vi "proc_checkErrors.vi"(1 "handle":i32) -> (0 "return value":i32)   [LabVIEW 2010]
uses:
  lib/MWT.dll
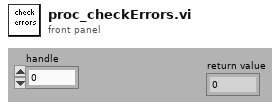
[diagram p1: front panel]
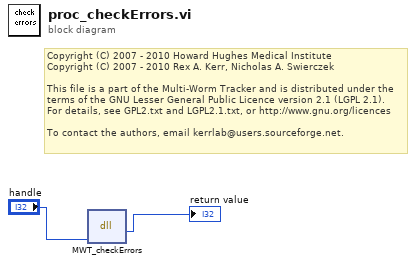
[diagram p0: block diagram]
diagram:
  # "Copyright (C) 2007 - 2010 Howard Hughes Medical Institute\nCopyright (C) 2007 - 2010 Rex A. Kerr, Nicholas A. Swierczek\n \nThis file is a part of the Multi-Worm Tracker and is distributed under the\nterms of the GNU Lesser General Public Licence version 2.1 (LGPL 2.1).\nFor details, see GPL2.txt and LGPL2.1.txt, or http://www.gnu.org/licences\n \nTo contact the authors, email kerrlab@users.sourceforge.net."
  n1 = dll-call lib="C:/MWT/lib/MWT.dll" fn="MWT_checkErrors"("handle"="handle") -> ("return type"=→"return value":i32)  [unwired: 4 in, 2 out]
